vi "RemoveCommentsFromStringArray.vi"(10 "comment prefix (%)":string="%", 11 "input text":string[](array[string])) -> (3 "output array":string[](array[string]))   [LabVIEW 2011]
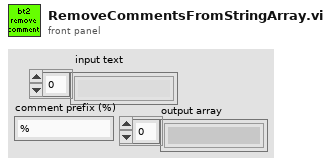
[diagram p1: front panel]
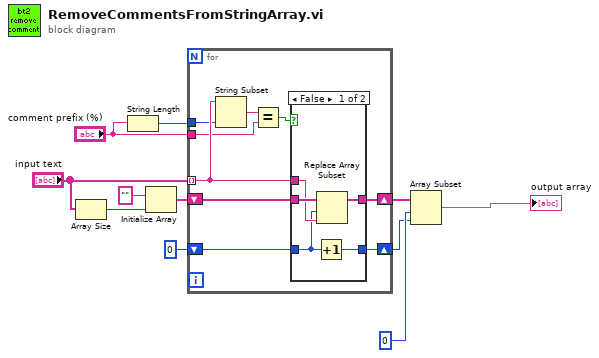
[diagram p0: block diagram]
diagram:
  n1 = Array Size(array="input text") -> (size(s)=w10:i32)
  n2 = String Length(string="comment prefix (%)") -> (length=w2:i32)
  n3 = Initialize Array("", w10) -> (w8:string[])
  n4 = for {
    tunnel: "input text" -> [w15] mode=indexing
    shift-right: [w17] -> w4
    shift-left: 0 -> [w18]
    shift-right: [w14] -> w6
    shift-left: w8 -> [w16]
    tunnel: w2 -> [w13]
    tunnel: "comment prefix (%)" -> [w12]
    n5 = String Subset(string=w15, length (rest)=w13) -> (substring=w20:string)  [unwired: 1 in]
    n6 = Equal?(x=w20, y=w12) -> (x = y?=w19:bool)
    n7 = case shown="False" w19 {
      tunnel: w18 -> [w23 w26]
      tunnel: [w22 w26] -> w17
      tunnel: w16 -> [w25 w27]
      tunnel: w15 -> [w24 _]
      tunnel: [w21 w27] -> w14
      frame False {
        n8 = Increment(x=w23) -> (x+1=w22:i32)
        n9 = Replace Array Subset(array=w25, new element=w24, index=w23) -> (w21:string[])
      }
      frame True {
      }
    }
  }
  n10 = Array Subset(array=w6, index=0, length=w4) -> (→"output array":string[])
